vi "WonKwangCam.vi"(4 "Number of Image Buffers":u32=2, 5 "Stop (F)":bool, 7 "error in":errorcluster) -> (20 "Image Out":T1(plugin-control), 21 "All Image Buffers Out":refnum<image>[](array[refnum]), 25 "Frame Rate":dbl, 26 "Stopped":bool, 27 "error out":errorcluster)   [LabVIEW 2011]
doc: "Creates, and edits acquisitions using the NI Vision Acquisition Express VI.\n\nThe NI Vision Acquisition Wizard is launched by placing the Express VI on the block diagram. Select an acquisition source and configure an acquisition using NI-IMAQ, NI-IMAQdx, or simulate an acquisition by reading an AVI or image files from a folder. After an acquisition is configured, select controls and indicators to be able to programmatically set in LabVIEW. Double-click the Vision Acquisition Express VI to edit the acquisition.\n\nNote: Any images created by the Express VI need to be disposed after use. Use the IMAQ Dispose.vi to cleanup the images output by the Express VI when they are no longer needed."
uses:
  <vilib>/vision/driver/NI_Vision_Acquisition_Software.lvlib
  C:/Program Files (x86)/National Instruments/LabVIEW 2011/resource/objmgr/imaqdx.rc
panel:
  in  "Gamma::Mode":u32(ring)=1 items=["Absolute"=1, "Relative"=0, "Off"=2, "Ignored"=5]
  in  "Gain::Value":dbl=24.00007438659668 min=-2.8151726722717285 max=12.0
  in  "Gain::Mode":u32(ring)=1 items=["Absolute"=1, "Auto"=3, "Relative"=0, "One Push"=4, "Ignored"=5]
  in  "Frame Rate::Value":dbl=60.0 min=1.0 max=60.0
  in  "Frame Rate::Mode":u32(ring)=1 items=["Absolute"=1, "Auto"=3, "Relative"=0, "Off"=2, "Ignored"=5]
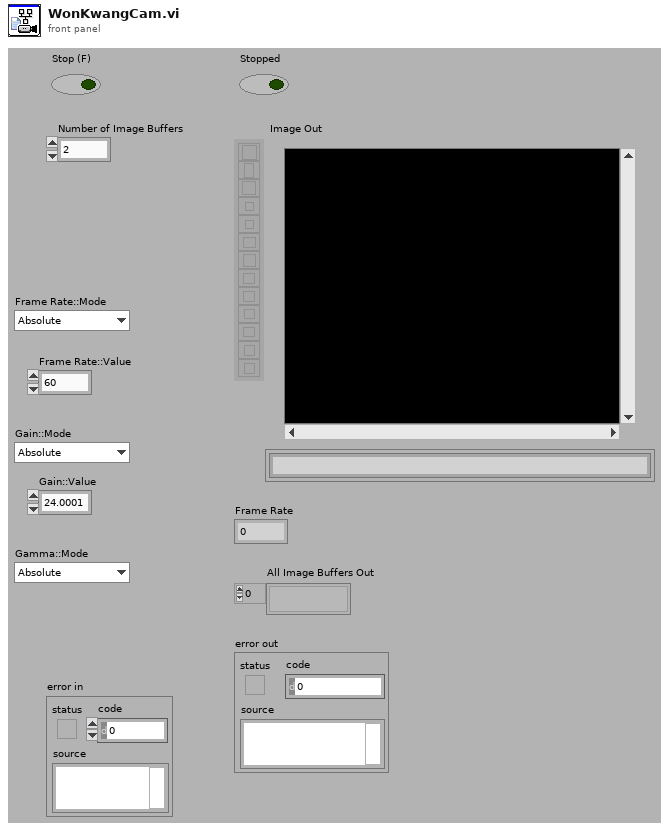
[diagram p1: front panel]
types:
  T1 = typedef "IMAQ Image.ctl" = refnum<image>
  T2 = typedef "IMAQdx.ctl" = refnum<k21>
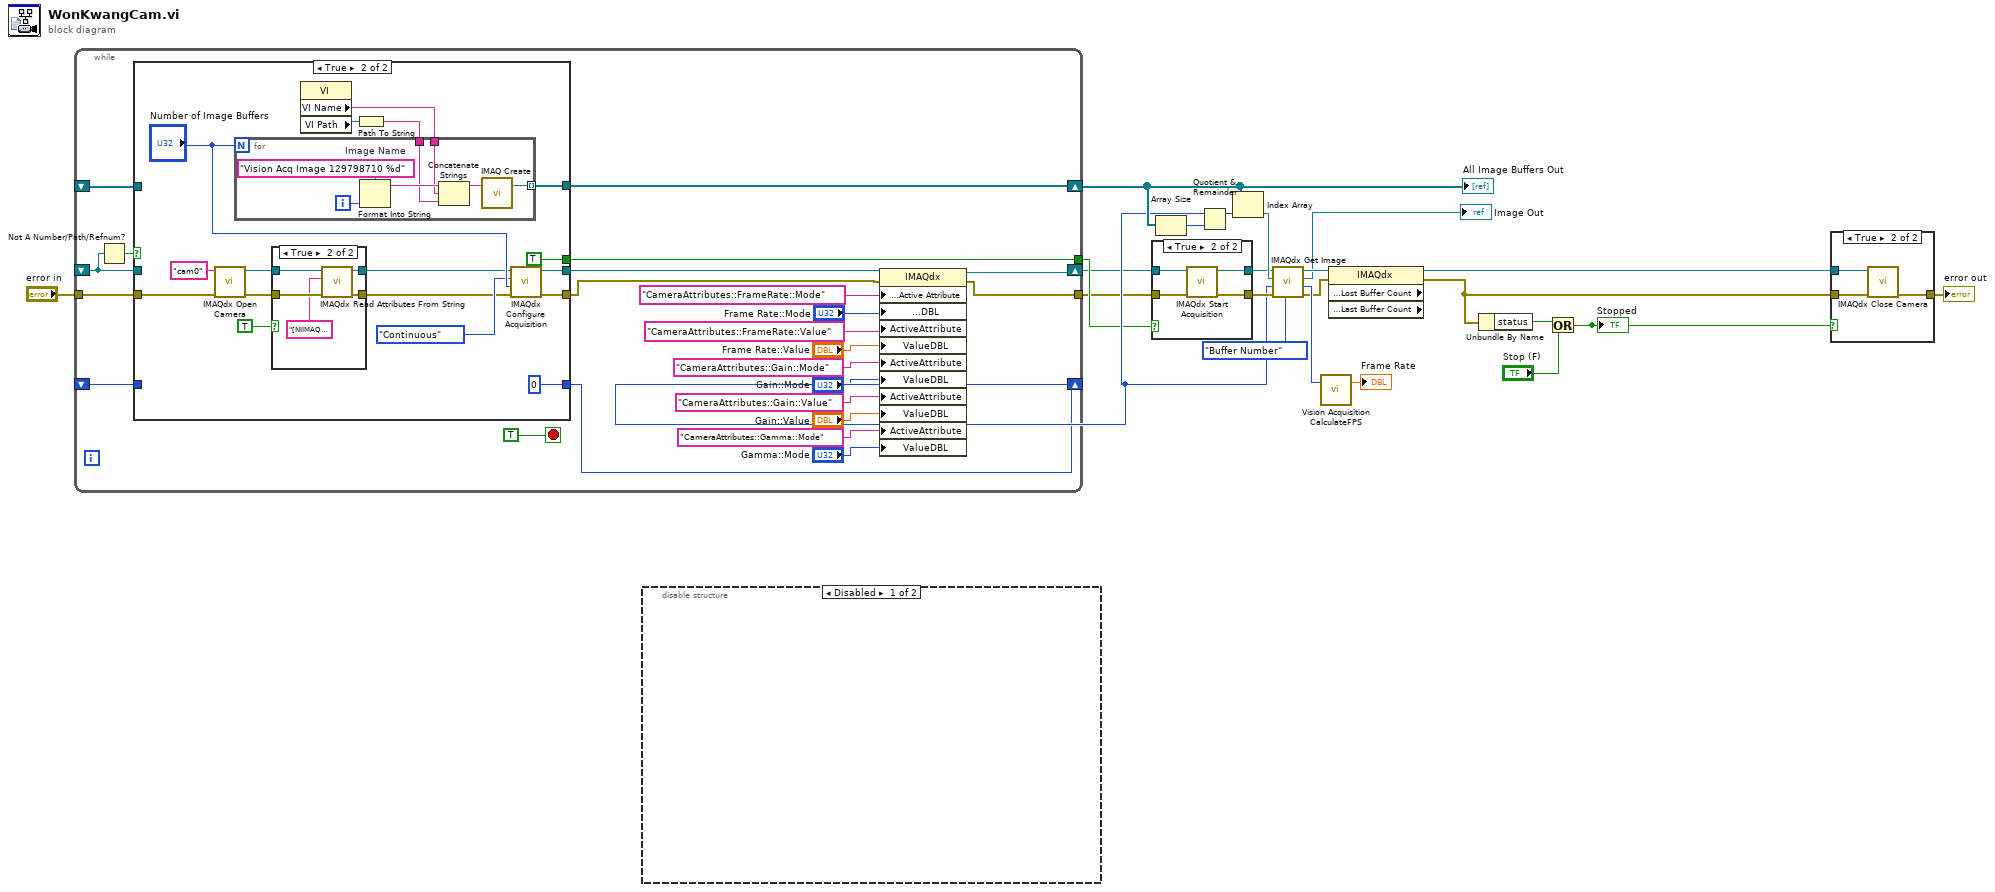
[diagram p0: block diagram]
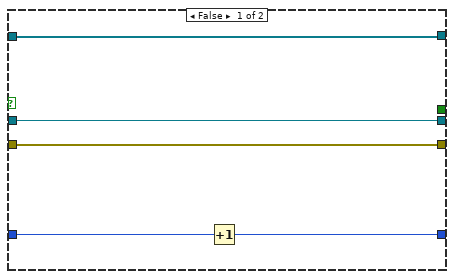
[diagram p5: hidden frame]
diagram:
  n1 = while {
    shift-right: [w25] -> w2
    shift-left: _ -> [w40]
    tunnel: [w24] -> w1
    tunnel: "error in" -> [w46]
    shift-right: [w44] -> w13
    shift-left: _ -> [w43]
    shift-right: [w42] -> w7
    shift-left: _ -> [w41]
    tunnel: [w38] -> w6
    stop <- TRUE stop-if-true
    n2 = Not A Number/Path/Refnum?(number/path/refnum=w40) -> (NaN/Path/Refnum?=w39:bool)
    n3 = case shown="True" w39 {
      tunnel: [w51 w66] -> w27
      tunnel: w40 -> [w51 _]
      tunnel: [w50 w65] -> w26
      tunnel: w46 -> [w50 w68]
      tunnel: [w49 w64] -> w44
      tunnel: w43 -> [w49 _]
      tunnel: [w47 0] -> w42
      tunnel: w41 -> [w48 _]
      tunnel: [_ TRUE] -> w38
      frame False {
        n4 = Increment(x=w48) -> (x+1=w47:i32)
      }
      frame True {
        n5 = call <vilib>:"IMAQdx Open Camera.vi"("error in"=w68, "Session In"="cam0" ("Interface Name")) -> ("error out"=w56:errorcluster, "Session Out"=w57:T2)  [unwired: 1 in, 7 out]
        n6 = case shown="True" TRUE ("Init Attributes") {
          tunnel: w57 -> [w70 w75]
          tunnel: w56 -> [w69 w74]
          tunnel: [w70 w73] -> w55
          tunnel: [w69 w72] -> w54
          frame False {
          }
          frame True {
            n7 = call <vilib>:"IMAQdx Read Attributes From String.vi"("error in"=w74, "Attributes String In"="[NIIMAQ_HEADER]\nType = 2\nVersion = 8\n\n[CAMERA_DATA]\nAcquisitionAttributes::VideoMode = \"640 x 480 Mono 8 120.00 fps\"\nAcquisitionAttributes::OffsetX = \"0\"\nAcquisitionAttributes::OffsetY = \"0\"\nAcquisitionAttributes::Width = \"640\"\nAcquisitionAttributes::Height = \"480\"\nAcquisitionAttributes::Bayer::GainB = \"1\"\nAcquisitionAttributes::Bayer::GainG = \"1\"\nAcquisitionAttributes::Bayer::GainR = \"1\"\nAcquisitionAttributes::Bayer::Pattern = \"Use hardware value\"\nAcquisitionAttributes::BitsPerPixel = \"10-bit\"\nAcquisitionAttributes::Controller::DesiredStreamChannel = \"0\"\nAcquisitionAttributes::Controller::StreamChannelMode = \"Automatic\"\nAcquisitionAttributes::IgnoreFirstFrame = \"false\"\nAcquisitionAttributes::OverwriteMode = \"Get Newest\"\nAcquisitionAttributes::PixelSignedness = \"Signed\"\nAcquisitionAttributes::ReceiveTimestampMode = \"None\"\nAcquisitionAttributes::ReserveDualPackets = \"true\"\nAcquisitionAttributes::ShiftPixelBits = \"true\"\nAcquisitionAttributes::Speed = \"800 Mbps\"\nAcquisitionAttributes::SwapPixelBytes = \"false\"\nAcquisitionAttributes::Timeout = \"5000\"\nCameraAttributes::AutoExposure::Mode = \"Auto\"\nCameraAttributes::Brightness::Mode = \"Absolute\"\nCameraAttributes::FrameRate::Mode = \"Absolute\"\nCameraAttributes::Gain::Mode = \"Absolute\"\nCameraAttributes::Gamma::Mode = \"Absolute\"\nCameraAttributes::Sharpness::Mode = \"Auto\"\nCameraAttributes::Shutter::Mode = \"Auto\"\nCameraAttributes::Temperature::Mode = \"UnknownEnumValue\"\nCameraAttributes::TriggerDelay::Mode = \"Off\"\nCameraAttributes::Brightness::Value = \"6.243896484375\"\nCameraAttributes::FrameRate::Value = \"120\"\nCameraAttributes::Gain::Value = \"24.00007438659668\"\nCameraAttributes::Gamma::Value = \"2.0048828125\"\nCameraAttributes::Temperature::Current = \"3084\"\nCameraAttributes::Temperature::Target = \"2931\"\nCameraAttributes::Trigger::TriggerMode = \"Off\"\nCameraAttributes::Trigger::TriggerActivation = \"Level Low\"\nCameraAttributes::Trigger::TriggerParameter = \"0\"\nCameraAttributes::Trigger::TriggerSource = \"Source 0\"\n" ("Attributes"), "Session In"=w75) -> ("error out"=w72:errorcluster, "Session Out"=w73:T2)  [unwired: 7 out]
          }
        }
        n8 = property class="VI"() -> ("VI Name"=w59:string, "VI Path"=w60:path)  [unwired: 2 in, 2 out]
        n9 = Path To String(path=w60) -> (string=w58:string)
        n10 = for "For Loop_template0" {
          N: "Number of Image Buffers" -> [_]
          tunnel: [w82] -> w64 mode=indexing
          tunnel: w59 -> [w77]
          tunnel: w58 -> [w76]
          i -> [w81]
          w80 = "Vision Acq Image 129798710 %d"  # Image Name
          n11 = Format Into String(format string=w80, w81) -> (resulting string=w79:string)  [unwired: 2 in, 1 out]
          n12 = Concatenate Strings(w79, w77, w76) -> (w78:string)
          n13 = call "IMAQ Create"("Image Name"=w78) -> ("New Image"=w82:T1)  [unwired: 3 in, 2 out]
        }
        n14 = call <vilib>:"IMAQdx Configure Acquisition.vi"("error in"=w54, "Number of Buffers"="Number of Image Buffers", "Continuous?"=enum32{"One Shot", "Continuous"}."Continuous" ("Mode"), "Session In"=w55) -> ("error out"=w65:errorcluster, "Session Out"=w66:T2)  [unwired: 6 out]
      }
    }
    n15 = property class="IMAQdx"(reference=w27, error in=w26, "Camera Attributes:Active Attribute"="CameraAttributes::FrameRate::Mode" ("Name"), "Camera Attributes:Value:DBL"="Frame Rate::Mode", "ActiveAttribute"="CameraAttributes::FrameRate::Value" ("Name"), "ValueDBL"="Frame Rate::Value", "ActiveAttribute"="CameraAttributes::Gain::Mode" ("Name"), "ValueDBL"="Gain::Mode", "ActiveAttribute"="CameraAttributes::Gain::Value" ("Name"), "ValueDBL"="Gain::Value", "ActiveAttribute"="CameraAttributes::Gamma::Mode" ("Name"), "ValueDBL"="Gamma::Mode") -> (reference out=w25:T2, error out=w24:errorcluster)
  }
  "All Image Buffers Out" <- w13
  n16 = disable-structure shown="Disabled" {
    frame Disabled {
    }
    frame Enabled {
    }
  }
  n17 = case shown="True" w6 {
    tunnel: w2 -> [w84 w88]
    tunnel: w1 -> [w83 w87]
    tunnel: [w83 w86] -> w8
    tunnel: [w84 w85] -> w9
    frame False {
    }
    frame True {
      n18 = call <vilib>:"IMAQdx Start Acquisition.vi"("error in"=w87, "Session In"=w88) -> ("error out"=w86:errorcluster, "Session Out"=w85:T2)  [unwired: 8 out]
    }
  }
  n19 = Array Size(array=w13) -> (size(s)=w14:i32)
  n20 = Quotient & Remainder(x=w7, y=w14) -> (x-y*floor(x/y)=w12:i32)  [unwired: 1 out]
  n21 = Index Array(array=w13, index=w12) -> (element=w11:T1)
  n22 = call <vilib>:"IMAQdx Get Image.vi"("Buffer Number Mode (Next)"=enum32{"Next", "Last", "Buffer Number"}."Buffer Number" ("Buffer Number Mode (Next)_template1"), "error in"=w8, "Buffer Number In"=w7, "Image In"=w11, "Session In"=w9) -> ("error out"=w16:errorcluster, "Buffer Number Out"=w20:u32, "Image Out"=→"Image Out":T1, "Session Out"=w17:T2)  [unwired: 3 out]
  n23 = call <vilib>:"Vision Acquisition CalculateFPS.vi"("buffer number"=w20) -> ("acquired FPS"=→"Frame Rate":dbl)  [unwired: 2 out]
  n24 = property class="IMAQdx" props=["Status Information:Lost Buffer Count", "Status Information:Last Buffer Count"](reference=w17, error in=w16) -> (reference out=w5:T2, error out=w10:errorcluster)  [unwired: 2 out]
  n25 = Unbundle By Name(w10) -> ("status"=w22:bool)
  n26 = Or(x=w22, y="Stop (F)") -> (x .or. y?=w4:bool)
  "Stopped" <- w4
  n27 = case "Case Structure_template1" shown="True" w4 {
    tunnel: [w89 w91] -> w3
    tunnel: w10 -> [w89 w92]
    tunnel: w5 -> [_ w90]
    frame False {
    }
    frame True {
      n28 = call <vilib>:"IMAQdx Close Camera.vi"("error in"=w92, "Session In"=w90) -> ("error out"=w91:errorcluster)  [unwired: 9 out]
    }
  }
  "error out" <- w3
